vi "全局 TCPIP超时.vi"() -> ()   [LabVIEW 2011]
panel:
  in  "超时":dbl
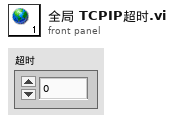
[diagram p1: front panel]
diagram:
